vi "GalvosStart.vi"(8 "error in (no error)":errorcluster, 11 "Microscope in":refnum<class "Microscope.lvclass">) -> (0 "error out":errorcluster, 3 "Microscope out":refnum<class "Microscope.lvclass">)   [LabVIEW 2012, in "Microscope.lvclass"]
uses:
  classes/Microscope.lvclass
  classes/Microscope.lvclass/Microscope.ctl
  <vilib>/DAQmx/write.llb/DAQmx Write (Analog 1D Wfm NChan NSamp).vi
  <vilib>/DAQmx/configure/timing.llb/DAQmx Timing (Sample Clock).vi
  <vilib>/DAQmx/configure/trigger.llb/DAQmx Start Trigger (Digital Edge).vi
  <vilib>/DAQmx/miscellaneous.llb/DAQmx Fill In Error Info.vi
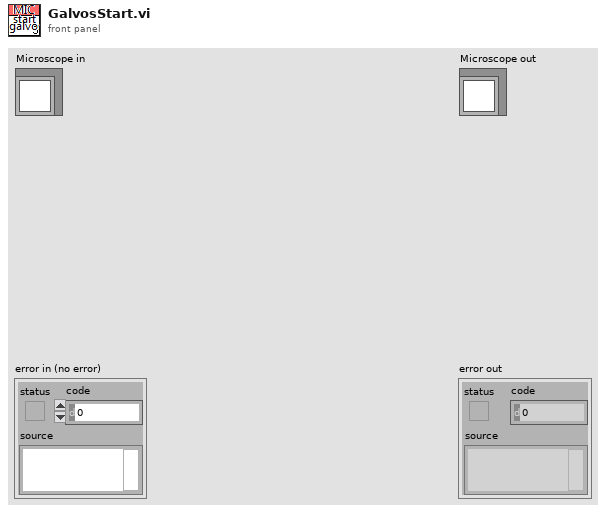
[diagram p1: front panel]
types:
  T1 = cluster{"x pixels":i32, "x voltage min":dbl, "x voltage max":dbl, "y pixels":i32, "y voltage min":dbl, "y voltage max":dbl, "x pts flyback":i32, "y pts flyback":i32, "Zoom":dbl}
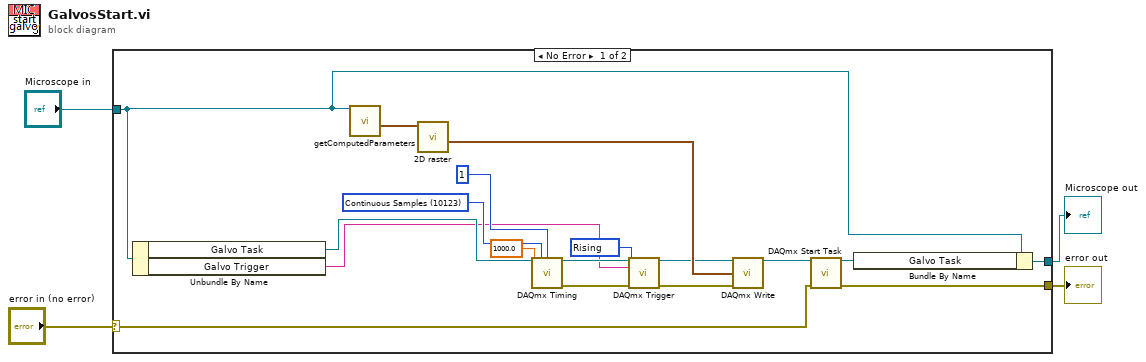
[diagram p0: block diagram]
diagram:
  n1 = case shown="No Error" "error in (no error)" {
    selector: "error in (no error)" -> [w19 w24]
    tunnel: [w21 w24] -> w3
    tunnel: [w22 w23] -> w1
    tunnel: "Microscope in" -> [w11 w23]
    frame No Error {
      w7 = 10280 items=["Rising"=10280, "Falling"=10171] ("edge")
      w12 = 10123 items=["Finite Samples"=10178, "Continuous Samples"=10123, "Hardware Timed Single Point"=12522] ("sample mode")
      n2 = Unbundle By Name(w11) -> ("Galvo Task"=w9:refnum<k21>, "Galvo Trigger"=w8:tag)
      n3 = call "getComputedParameters.vi"("Microscope in"=w11) -> ("Scanning Parameters"=w6:T1)  [unwired: 11 in, 3 out]
      n4 = call "2D raster.vi"("Scanning Parameters"=w6) -> ("X and Y"=w15:waveform(dbl)[])  [unwired: 8 in, 2 out]
      n5 = call-poly <vilib>:"DAQmx Timing.vi"("task/channels in"=w9, "sample mode"=w12, "samples per channel"=1, "rate"=1000.0) -> ("task out"=w13:refnum<k21>, "error out"=w16:errorcluster)  [unwired: 10 in]
      n6 = call-poly <vilib>:"DAQmx Trigger.vi"("task/channels in"=w13, "source"=w8, "edge"=w7, "error in"=w16) -> ("task out"=w14:refnum<k21>, "error out"=w17:errorcluster)  [unwired: 10 in]
      n7 = call-poly <vilib>:"DAQmx Write.vi"("task/channels in"=w14, "data"=w15, "error in"=w17) -> ("task out"=w10:refnum<k21>)  [unwired: 10 in, 2 out]
      n8 = call <vilib>:"DAQmx Start Task.vi"("task/channels in"=w10, "error in"=w19) -> ("task out"=w20:refnum<k21>, "error out"=w21:errorcluster)  [unwired: 12 in]
      n9 = Bundle By Name(cluster=w11, "Galvo Task"=w20) -> (w22:refnum<class "Microscope.lvclass">)
    }
    frame Error {
    }
  }
  "error out" <- w3
  "Microscope out" <- w1
